vi "PREP FIELD.vi"(6 "Numeric":i32, 7 "Lead- Mode Ramp Rate (A/s)":dbl, 9 "PSU Status In":T1 {"Trip Current" format="%.3f"; "Trip Field" format="%.4f"; "Voltage" format="%.2f"; "Field Constant" format="%.6f"; "MID Setpoint (T)" format="%.4f"; "MID Setpoint (A)" format="%.3f"; "MAX Setpoint (T)" format="%.4f"; "MAX Setpoint (A)" format="%.3f"; "Heater Voltage" format="%.2f"; "V Limit (V)" format="%.2f"; "Ramp Rate (A/s)" format="%.3f"; "Output (A)" format="%.3f"; "Output (T)" format="%.4f"; "Persistent Current" format="%.3f"; "Persistent Field" format="%.4f"}, 10 "MagQ in":refnum<queue>, 11 "VISA Refnum in":refnum<visa-resource-name>) -> (0 "error out":errorcluster, 1 "Output (T)":dbl, 2 "MagQ out":refnum<queue>, 3 "VISA Refnum out":refnum<visa-resource-name>)   [LabVIEW 2025]
uses:
  <instrlib>/SMS LabVIEW Drivers/Source Code/Cryogenic Ltd SMSXXX.lvlib
  <instrlib>/SMS LabVIEW Drivers/Source Code/Public/PSU Status.ctl
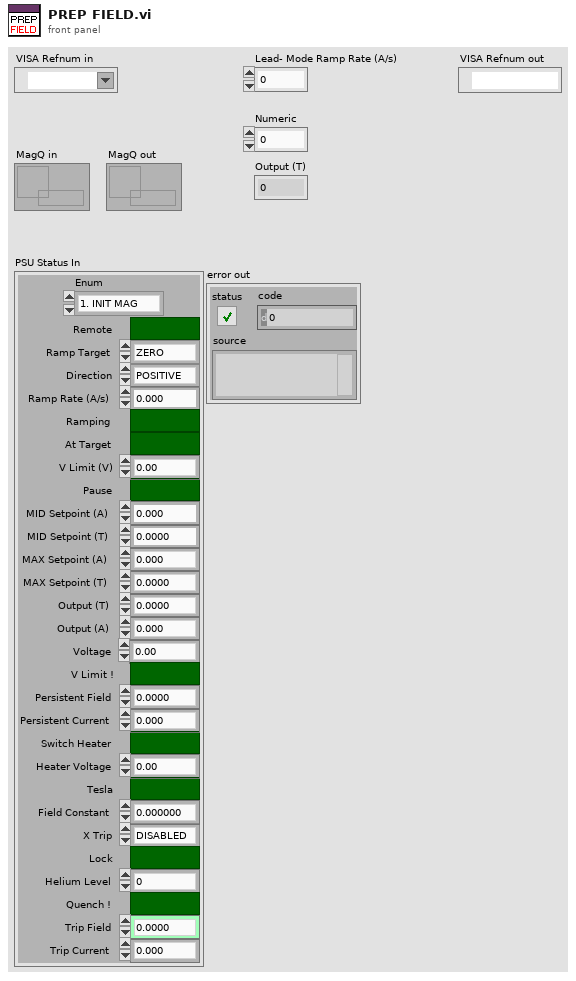
[diagram p1: front panel]
types:
  T1 = typedef "Cryogenic Ltd SMSXXX.lvlib/PSU Status.ctl" = cluster{"Ramp Target":enum16{"ZERO", "MID", "MAX"}, "Pause":bool, "Switch Heater":bool, "Persistent Field":dbl, "Persistent Current":dbl, "Tesla":bool, "Output (T)":dbl, "Output (A)":dbl, "X Trip":enum16{"DISABLED", "ENABLED", "ACTIVE"}, "Ramp Rate (A/s)":dbl, "V Limit (V)":dbl, "Heater Voltage":dbl, "MAX Setpoint (A)":dbl, "MAX Setpoint (T)":dbl, "MID Setpoint (A)":dbl, "MID Setpoint (T)":dbl, "Lock":bool, "Field Constant":dbl, "Remote":bool, "Direction":enum16{"POSITIVE", "NEGATIVE", "OPEN", "UNIPOLAR"}, "Helium Level":u16, "Quench !":bool, "Voltage":dbl, "V Limit !":bool, "Ramping":bool, "At Target":bool, "Trip Field":dbl, "Trip Current":dbl, "Enum":enum16{"1. INIT MAG", "2. MAG ON ", "3. MAG_STAB", "4. MAG IDLE", "5. NEXT FIELD", "6. MAG OFF (Reset)"}}
  T2 = enum16{"RAMP TO ZERO", "RAMP TO MID", "RAMP TO MAX"}
  T3 = enum16{"1. INIT MAG", "2. MAG ON", "3. MAG_STAB", "4. MAG IDLE", "5. PREP NEXT FIELD", "6. APPLY NEXT FIELD", "7. PREP OFF", "8. MAG OFF (Reset)"}
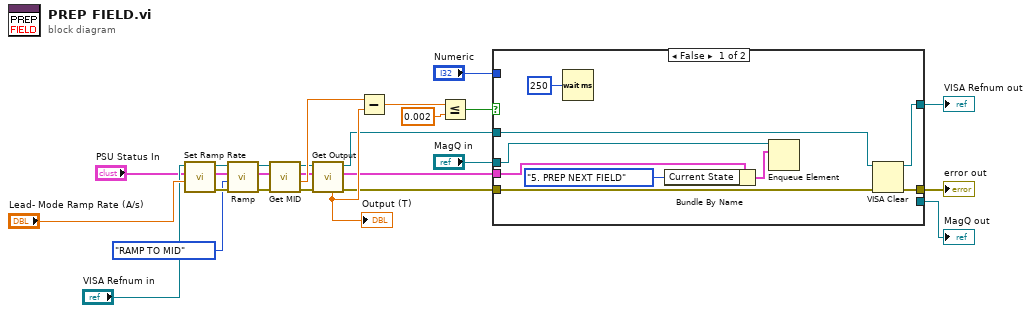
[diagram p0: block diagram]
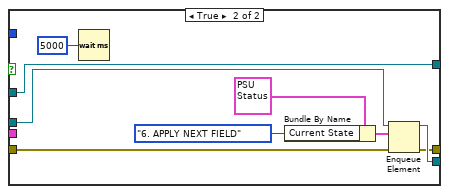
[diagram p2: hidden frame]
diagram:
  n1 = call <instrlib>:"Set Ramp Rate.vi"("Ramp Rate (A/s)"="Lead- Mode Ramp Rate (A/s)", "PSU Status In"="PSU Status In", "VISA Resource Name In"="VISA Refnum in") -> ("Error out"=w15:errorcluster, "PSU Status Out"=w16:T1, "VISA Resource Name Out"=w14:refnum<visa-resource-name>)  [unwired: 5 in, 1 out]
  n2 = call <instrlib>:"Ramp.vi"("Error in (no error)"=w15, "Ramp Target"=T2."RAMP TO MID", "PSU Status In"=w16, "VISA Resource Name In"=w14) -> ("Error out"=w3:errorcluster, "PSU Status Out"=w4:T1, "VISA Resource Name Out"=w2:refnum<visa-resource-name>)  [unwired: 4 in, 1 out]
  n3 = call <instrlib>:"Get MID.vi"("Error in (no error)"=w3, "PSU Status In"=w4, "VISA Resource Name In"=w2) -> ("Error out"=w9:errorcluster, "MID Setpoint (T)"=w22:dbl, "PSU Status Out"=w7:T1, "VISA Resource Name Out"=w8:refnum<visa-resource-name>)  [unwired: 3 in, 2 out]
  n4 = call <instrlib>:"Get Output.vi"("Error in (no error)"=w9, "PSU Status In"=w7, "VISA Resource Name In"=w8) -> ("Error out"=w11:errorcluster, "PSU Status Out"=w12:T1, "VISA Resource Name Out"=w10:refnum<visa-resource-name>, "Output (T)"=w26:dbl)  [unwired: 3 in, 2 out]
  "Output (T)" <- w26
  n5 = Subtract(x=w22, y=w26) -> (x-y=w23:dbl)
  n6 = Less Or Equal?(x=w23, y=0.002) -> (x <= y?=w25:bool)
  n7 = case shown="False" w25 {
    tunnel: w11 -> [w33 w39]
    tunnel: "Numeric" -> [_ _]
    tunnel: [_ w44] -> w6
    tunnel: w10 -> [w34 w37]
    tunnel: w12 -> [w29 _]
    tunnel: "MagQ in" -> [w30 w42]
    tunnel: [w31 w38] -> w20
    tunnel: [w32 w37] -> w21
    frame False {
      n8 = Wait (ms)(milliseconds to wait=u32 250) -> ()  [unwired: 1 out]
      n9 = Bundle By Name(cluster=w29, "Current State"=T3."5. PREP NEXT FIELD") -> (w28:T1)
      n10 = Enqueue Element(queue=w30, element=w28) -> ()  [unwired: 2 in, 3 out]
      n11 = VISA Clear(VISA resource name=w34, error in (no error)=w33) -> (VISA resource name out=w32:refnum<visa-resource-name>, error out=w31:errorcluster)
    }
    frame True {
      n12 = Wait (ms)(milliseconds to wait=u32 5000) -> ()  [unwired: 1 out]
      n13 = Bundle By Name(cluster=T1 {"Ramp Target"=enum."ZERO", "Pause"=FALSE, "Switch Heater"=FALSE, "Persistent Field"=0.0, "Persistent Current"=0.0, "Tesla"=FALSE, "Output (T)"=0.0, "Output (A)"=0.0, "X Trip"=enum."DISABLED", "Ramp Rate (A/s)"=0.0, "V Limit (V)"=0.0, "Heater Voltage"=0.0, "MAX Setpoint (A)"=0.0, "MAX Setpoint (T)"=0.0, "MID Setpoint (A)"=0.0, "MID Setpoint (T)"=0.0, "Lock"=FALSE, "Field Constant"=0.0, "Remote"=FALSE, "Direction"=enum."POSITIVE", "Helium Level"=0, "Quench !"=FALSE, "Voltage"=0.0, "V Limit !"=FALSE, "Ramping"=FALSE, "At Target"=FALSE, "Trip Field"=0.0, "Trip Current"=0.0, "Enum"=enum."1. INIT MAG"} ("PSU Status In"), "Current State"=T3."6. APPLY NEXT FIELD") -> (w41:T1)
      n14 = Enqueue Element(queue=w42, element=w41, error in (no error)=w39) -> (queue out=w44:refnum<queue>, error out=w38:errorcluster)  [unwired: 1 in, 1 out]
    }
  }
  "VISA Refnum out" <- w21
  "error out" <- w20
  "MagQ out" <- w6
